vi "Get Created Attributes.vi"(10 "Alias":string, 11 "TEMPLATE Actor in":refnum<class "TEMPLATE Actor.lvclass">) -> (1 "Is Found":bool, 2 "Created Attributes":refnum<class "Attributes.lvclass">)   [LabVIEW 2020, in "_Template.lvlib" / "Templates.lvlib" / "TEMPLATE Actor.lvlib" / "TEMPLATE Actor.lvclass"]
uses:
  TEMPLATE Actor.lvclass
  jettl/jettl/Actor/Actor/Actor.lvclass
  jettl/jettl/Attributes/Attributes/Attributes.lvclass
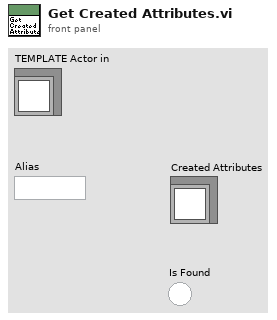
[diagram p1: front panel]
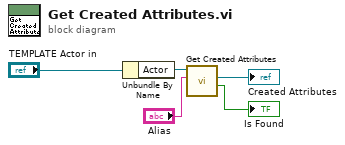
[diagram p0: block diagram]
diagram:
  n1 = Unbundle By Name("TEMPLATE Actor in") -> ("Actor"=w4:refnum<class "Actor.lvclass">)
  n2 = call-dynamic "Get Created Attributes.vi"("Alias"="Alias", "Actor in"=w4) -> ("Is Found"=→"Is Found":bool, "Created Attributes"=→"Created Attributes":refnum<class "Attributes.lvclass">)  [unwired: 8 in]
